vi "Test Replace Symbol.vi"(8 "error in (no error)":errorcluster, 11 "Test Case In":refnum<class "Conditional Disabled Configurator Test.lvclass">) -> (0 "error out":errorcluster, 3 "Test Case Out":refnum<class "Conditional Disabled Configurator Test.lvclass">)   [LabVIEW 2020, in "Conditional Disabled Configurator Test.lvclass"]
uses:
  Conditional Disabled Configurator Test.lvclass
  Conditional Disabled Configurator Test.lvclass/Conditional Disabled Configurator Test.ctl
  01074fa8-ee8a-411d-bc8b-fc92c4f90959.vi
  source/Conditional Disabled Configurator/Conditional Disabled Configurator.lvclass
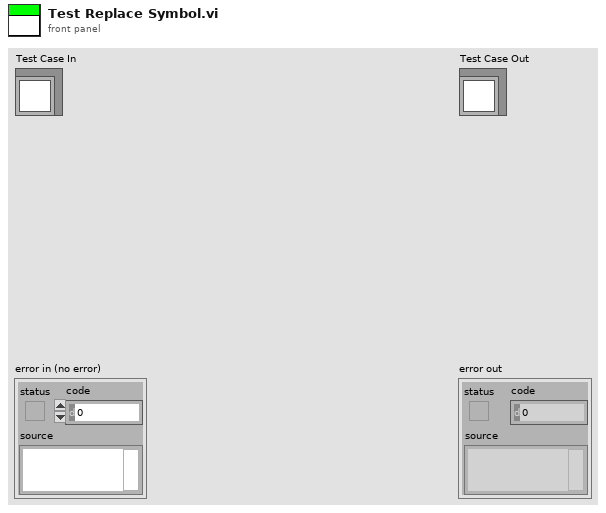
[diagram p1: front panel]
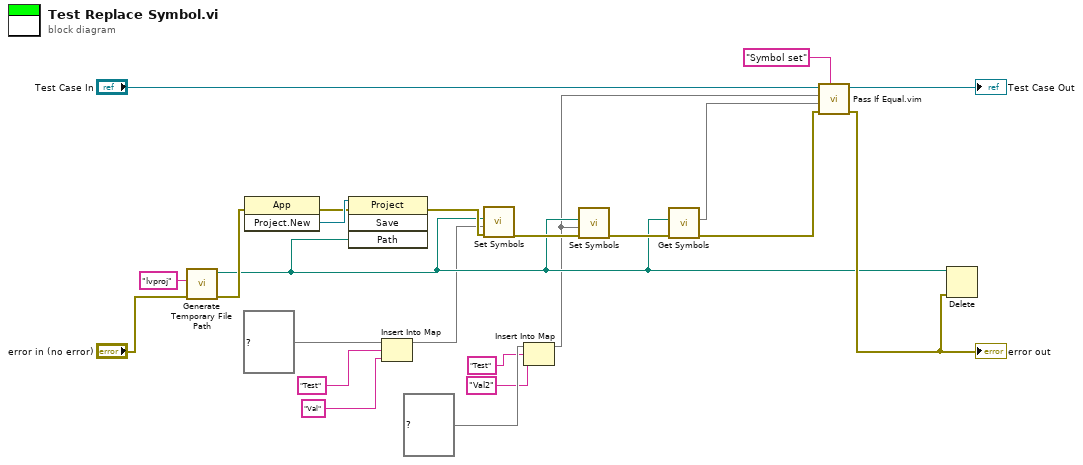
[diagram p0: block diagram]
diagram:
  n1 = call <vilib>:"Generate Temporary File Path.vi"("error in (no error)"="error in (no error)", "Temporary File Extension (tmp)"="lvproj") -> ("error out"=w19:errorcluster, "Unique Temporary File Path"=w3:path)  [unwired: 8 in]
  n2 = invoke class="App" method="Project.New"(error in=w19) -> (error out=w17:errorcluster, "Project:New"=w18:refnum<vi>)  [unwired: 2 in, 1 out]
  n3 = invoke class="Project" method="Save"(reference=w18, error in=w17, "Path"=w3) -> (error out=w16:errorcluster)  [unwired: 1 in, 3 out]
  n4 = Insert Into Map(map in=map{string, string} {} ("Symbols"), key="Test", value="Val") -> (map out=w1:map{string, string})  [unwired: 2 out]
  n5 = call "Set Symbols.vi"("error in (no error)"=w16, "Symbols"=w1, "Project Path"=w3) -> ("error out"=w8:errorcluster)  [unwired: 8 in]
  n6 = Insert Into Map(map in=map{string, string} {} ("Symbols"), key="Test", value="Val2") -> (map out=w2:map{string, string})  [unwired: 2 out]
  n7 = call "Set Symbols.vi"("error in (no error)"=w8, "Symbols"=w2, "Project Path"=w3) -> ("error out"=w7:errorcluster)  [unwired: 8 in]
  n8 = call "Get Symbols.vi"("error in (no error)"=w7, "Project Path"=w3) -> ("error out"=w11:errorcluster, "Symbols"=w12:map{string, string})  [unwired: 8 in]
  n9 = call "Pass If Equal.vim"("Description"="Symbol set", "error in (no error)"=w11, "Actual"=w12, "Expected"=w2, "LUnit Test Case In"="Test Case In") -> ("error out"=w9:errorcluster, "LUnit Test Case Out"=→"Test Case Out":refnum<class "Conditional Disabled Configurator Test.lvclass">)  [unwired: 5 in]
  "error out" <- w9
  n10 = Delete(path (use dialog)=w3, error in=w9) -> ()  [unwired: 3 in, 3 out]
